vi "SinglePlaneScan.vi"(0 "Sweep Time (µS)":u32 step=2, 1 "Phase Shift (µS)":i32(slide) scale=-1000.0..1000.0, 2 "Sweep Interval (µS)":u32 step=2, 3 "Sample Rate (kHz)":u32, 4 "Offset":dbl, 5 "Amplitude":dbl) -> ()   [LabVIEW 2013]
doc: "I. Description:\nThis example demonstrates how to continuously acquire and generate data at the same time, synchronized with one another.\n\nII. Instructions for Running:\n1. Select the physical channel to correspond to where your signal is input on the DAQ device. Also, select the corresponding channel for where your signal is being generated.\n2. Enter the minimum and maximum voltage ranges.\nNote: For better accuracy try to match the input range to the expected voltage level of the measured signal.\n3. Set the sample rate of the acquisition.\nNote: The rate should be at least twice as fast as the maximum frequency component of the signal being acquired. \n6. Select the Rate for the generation\n7. Select what type of signal to generate and the amplitude.\nNote: This example requires two DMA channels to run. If your hardware does not support two DMA channels, you need to set the Data Transfer Mechanism property for the Analog Output Task to use \"Interrupts\". The Data Transfer Mechanism property is located in the DAQmx Channel Property hierarchy at:\n\nDAQmx Channel Property Node>>Analog Output>>General Properties>>Advanced>>Data Transfer and Memory>>Data Transfer Mechanism\n\nRefer to your device documentation to determine how many DMA channels are supported for your hardware.\n\nIII. Block Diagram Steps:\n1. Create an analog input voltage channel. Also, create an analog output voltage channel.\n2. Set the rate for the sample clock. Additionally, define the sample mode to be continuous. Also, set the sample clock rate for the signal generation.\n2a. Call the Get Terminal Name with Device Prefix VI. This will take a Task and a terminal and create a properly formatted device + terminal name to use as the source of the Trigger.\n3. Define the parameters for a Digital Edge Start Trigger. Set the Analog output to trigger off the AI Start Trigger. This is an internal trigger signal.\n4. Use the Basic Function Generator VI to create the signal to be generated.\n5. Call the Start VI to arm the two functions. Make sure the analog output is armed before the analog input. This will ensure both will start at the same time.\n6. Read the waveform data in a loop until the user hits the stop button or an error occurs. The Is Task Done? VI is used to check for errors in the Analog Output Task.\n7. Call the Clear VI to Clear the Task\n8. Use the popup dialog box to display an error if any.\n\nIV. I/O Connections Overview:\nMake sure your signal input/output terminals match the Physical Channel I/O controls."
uses:
  <vilib>/Utility/error.llb/DialogType.ctl
  <vilib>/DAQmx/write.llb/DAQmx Write (Analog Wfm 1Chan NSamp).vi
  <vilib>/DAQmx/write.llb/DAQmx Write (Digital 1D Wfm NChan NSamp).vi
  <vilib>/DAQmx/create/channels.llb/DAQmx Create Channel (CO-Pulse Generation-Time).vi
  <vilib>/DAQmx/create/channels.llb/DAQmx Create Channel (AO-Voltage-Basic).vi
  <vilib>/DAQmx/configure/timing.llb/DAQmx Timing (Sample Clock).vi
  <vilib>/DAQmx/create/channels.llb/DAQmx Create Channel (DO-Digital Output).vi
  <vilib>/DAQmx/configure/trigger.llb/DAQmx Start Trigger (Digital Edge).vi
  <vilib>/DAQmx/miscellaneous.llb/DAQmx Fill In Error Info.vi
  <vilib>/Waveform/DWDTOps.llb/DWDT Uncompress Digital.vi
panel:
  out "AOTF":digitalwaveform(graph)
  out "Resolution (µS)":u32
  out "Number of Samples":u32
  out "CAMERA EXPOSURE TRIGGER":digitalwaveform(graph)
  out "MIRROR":waveform(dbl)(graph)
  # "For instructions, select Help>>Show Context Help"
  # "Output Channel Parameters"
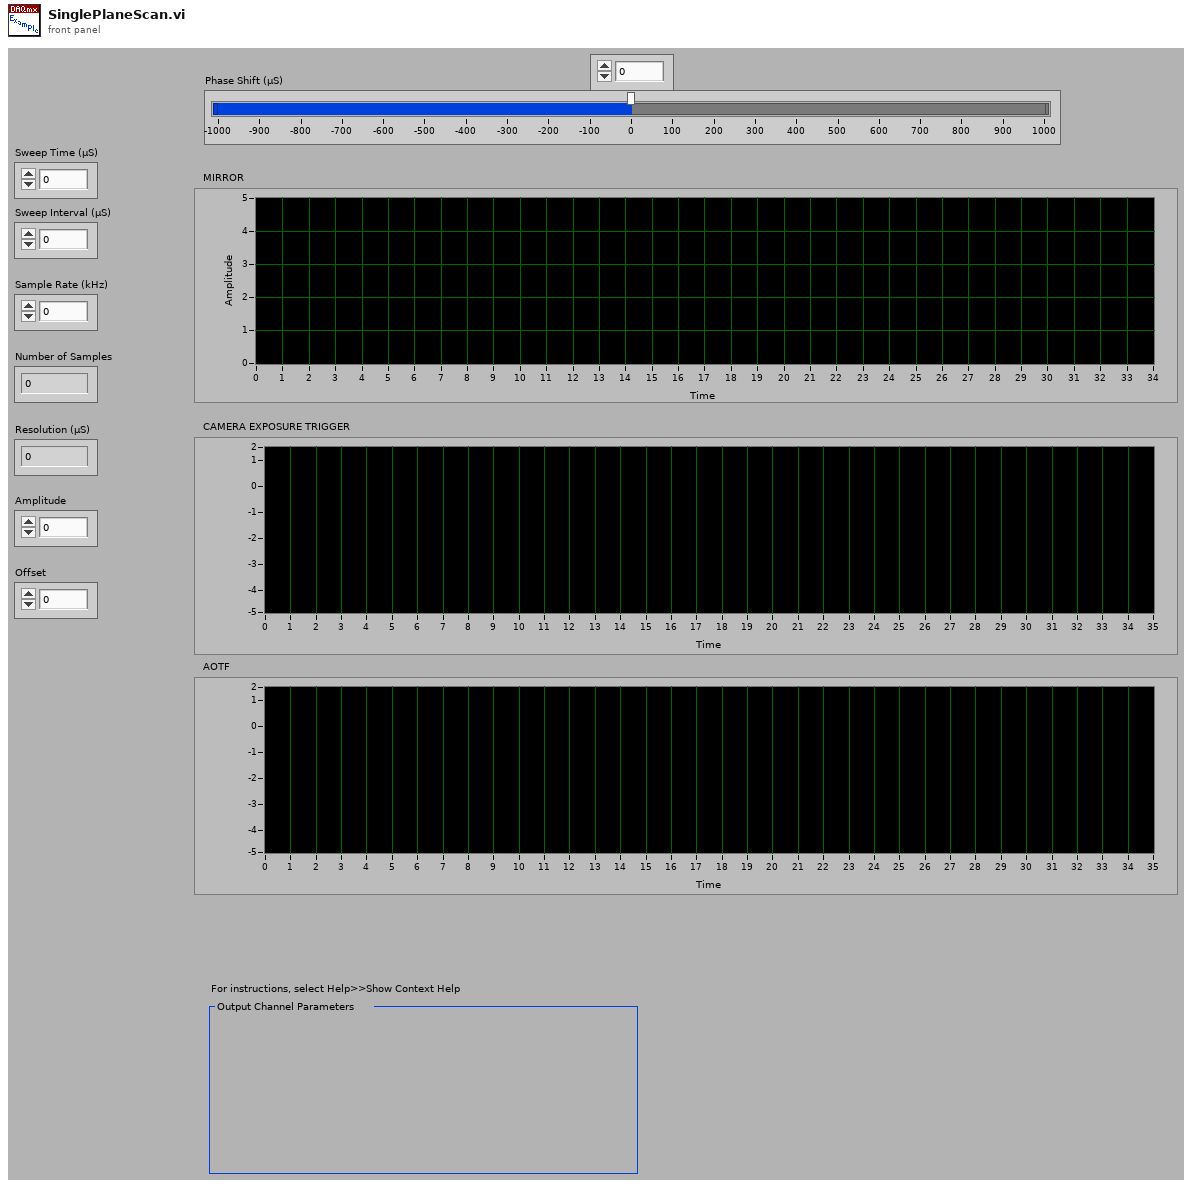
[diagram p1: front panel]
types:
  T1 = typedef "DialogType.ctl" = u16
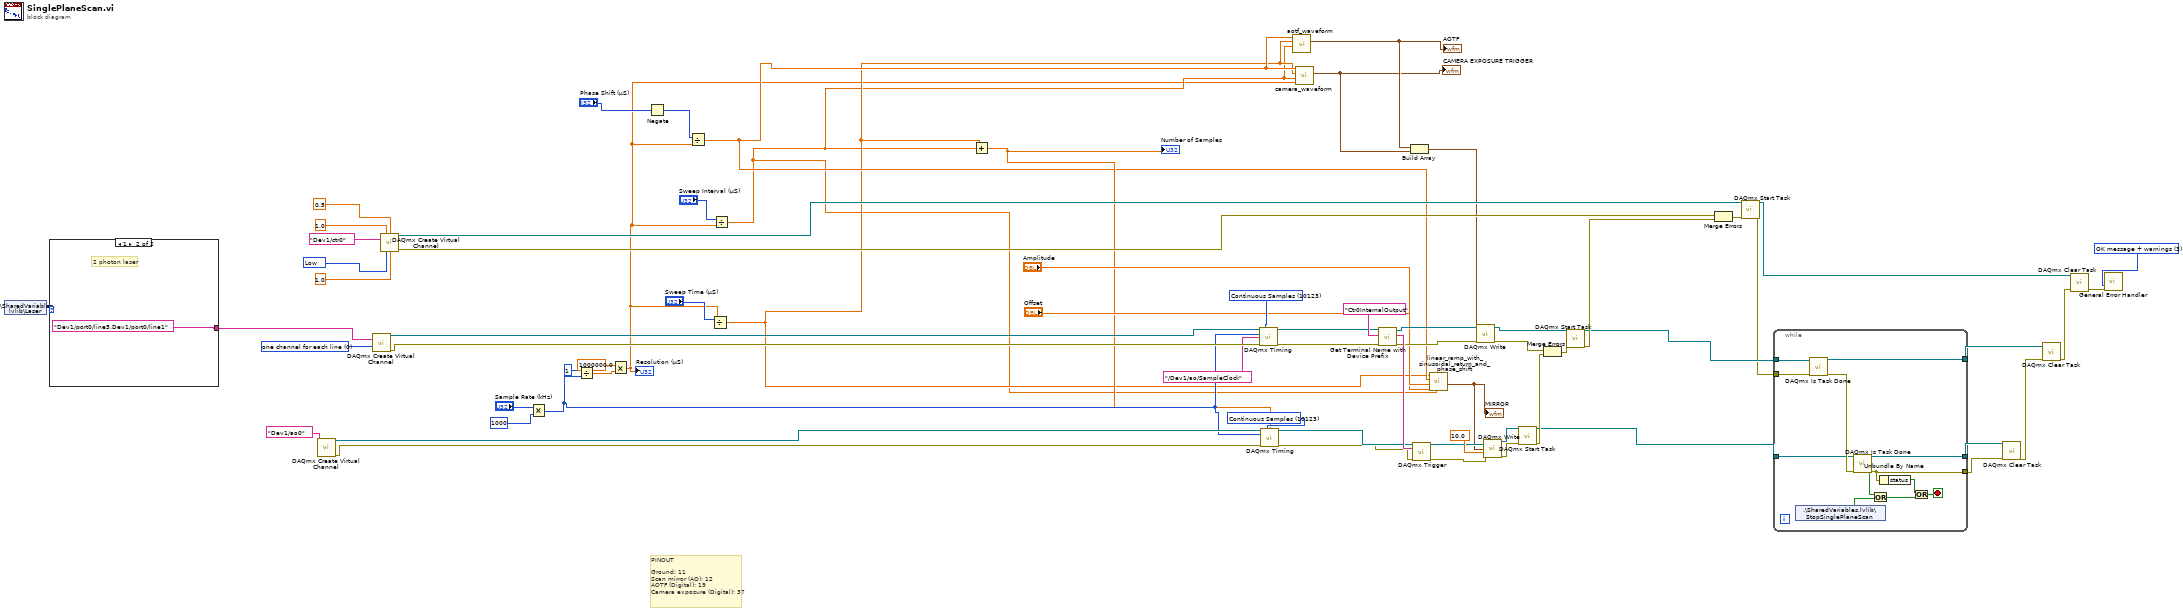
[diagram p0: block diagram]
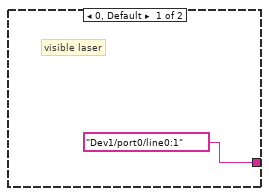
[diagram p2: hidden frame]
diagram:
  w25 = 0 items=["one channel for each line", "one channel for all lines"] ("line grouping")
  w36 = T1 3 items=["no dialog", "OK message", "continue or stop message", "OK message + warnings", "continue/stop + warnings"] ("type of dialog (OK msg:1)")
  w49 = 10214 items=["High"=10192, "Low"=10214] ("Idle State")
  w66 = 10123 items=["Finite Samples"=10178, "Continuous Samples"=10123] ("sample mode")
  w69 = 10123 items=["Finite Samples"=10178, "Continuous Samples"=10123] ("sample mode")
  # "PINOUT\n\nGround: 11\nScan mirror (AO): 12\nAOTF (Digital): 19\nCamera exposure (Digital): 37"
  n1 = shared-variable ".\\SharedVariables.lvlib\\Laser"() -> (w5:u8)  [unwired: 1 in, 1 out]
  n2 = case shown="1" w5 {
    tunnel: [tag "Dev1/port0/line0:1" ("Physical Channel") tag "Dev1/port0/line5,Dev1/port0/line1" ("Physical Channel")] -> w4
    frame 0, Default {
      # "visible laser"
    }
    frame 1 {
      # "2 photon laser"
    }
  }
  n3 = call-poly <vilib>:"DAQmx Create Virtual Channel.vi"("physical channels"=tag "Dev1/ao0") -> ("task out"=w65:refnum<k21>, "error out"=w64:errorcluster)  [unwired: 8 in, 5 out]
  n4 = call-poly <vilib>:"DAQmx Create Virtual Channel.vi"("lines"=w4, "line grouping"=w25) -> ("task out"=w67:refnum<k21>, "error out"=w68:errorcluster)  [unwired: 5 in, 7 out]
  n5 = call-poly <vilib>:"DAQmx Create Virtual Channel.vi"("high time"=1.0 ("High Time"), "low time"=0.5 ("Low Time"), "counter"=tag "Dev1/ctr0" ("Counter(s)"), "idle state"=w49, "initial delay"=1.0 ("Initial Delay")) -> ("task out"=w44:refnum<k21>, "error out"=w42:errorcluster)  [unwired: 4 in, 5 out]
  n6 = Multiply(x="Sample Rate (kHz)", y=u32 1000) -> (x*y=w15:u32)
  n7 = Divide(x=u32 1, y=w15) -> (x/y=w16:dbl)
  n8 = Multiply(x=1000000.0, y=w16) -> (x*y=w1:dbl)
  "Resolution (µS)" <- w1
  n9 = Negate(x="Phase Shift (µS)") -> (-x=w3:i32)
  n10 = Divide(x=w3, y=w1) -> (x/y=w10:dbl)
  n11 = Divide(x="Sweep Time (µS)", y=w1) -> (x/y=w9:dbl)
  n12 = Divide(x="Sweep Interval (µS)", y=w1) -> (x/y=w8:dbl)
  n13 = Add(x=w9, y=w8) -> (x+y=w12:dbl)
  "Number of Samples" <- w12
  n14 = call-poly <vilib>:"DAQmx Timing.vi"("task/channels in"=w67, "sample mode"=w69, "rate"=w15, "source"=tag "/Dev1/ao/SampleClock", "error in"=w68) -> ("task out"=w22:refnum<k21>, "error out"=w21:errorcluster)  [unwired: 2 in, 7 out]
  n15 = call-poly <vilib>:"DAQmx Timing.vi"("task/channels in"=w65, "sample mode"=w66, "samples per channel"=w12, "rate"=w15, "error in"=w64) -> ("task out"=w24:refnum<k21>, "error out"=w23:errorcluster)  [unwired: 2 in, 7 out]
  n16 = call "aotf_waveform.vi"("Sweep Interval (µS)"=w8, "Actual Sweep Time (µS)"=w9, "Phase Shift (µS)"=w10) -> ("Digital Waveform Graph"=w7:digitalwaveform)  [unwired: 8 in]
  "AOTF" <- w7
  n17 = call "camera_waveform.vi"("Resolution"=w1, "Sweep Interval (µS)"=w8, "Actual Sweep Time (µS)"=w9, "Phase Shift (µS)"=w10) -> ("Digital Waveform Graph"=w6:digitalwaveform)  [unwired: 7 in]
  "CAMERA EXPOSURE TRIGGER" <- w6
  n18 = call "Get Terminal Name with Device Prefix.vi"("error in (no error)"=w21, "Local Terminal Name"="Ctr0InternalOutput" ("terminal"), "task/channels in"=w22) -> ("error out"=w52:errorcluster, "Terminal Name with Device Prefix"=w57:tag, "task out"=w53:refnum<k21>)  [unwired: 1 in, 5 out]
  n19 = Build Array(w7, w6) -> (w26:digitalwaveform[])
  n20 = call-poly <vilib>:"DAQmx Trigger.vi"("task/channels in"=w24, "source"=w57, "error in"=w23) -> ("task out"=w59:refnum<k21>, "error out"=w60:errorcluster)  [unwired: 2 in, 9 out]
  n21 = call "linear_ramp_with_sinusoidal_return_and_phase_shift.vi"("Sweep Interval (µS)"=w8, "Offset"="Offset", "Amplitude"="Amplitude", "Phase Shift (µs)"=w10, "Sweep Time (µs)"=w9) -> ("Waveform Chart"=w27:waveform(dbl))  [unwired: 6 in]
  "MIRROR" <- w27
  n22 = call-poly <vilib>:"DAQmx Write.vi"("task/channels in"=w53, "data"=w26, "error in"=w52) -> ("task out"=w50:refnum<k21>, "error out"=w51:errorcluster)  [unwired: 2 in, 9 out]
  n23 = call-poly <vilib>:"DAQmx Write.vi"("task/channels in"=w59, "data"=w27, "timeout"=10.0 ("Wirite Timeout"), "error in"=w60) -> ("task out"=w62:refnum<k21>, "error out"=w61:errorcluster)  [unwired: 1 in, 9 out]
  n24 = call <vilib>:"DAQmx Start Task.vi"("task/channels in"=w62, "error in"=w61) -> ("task out"=w31:refnum<k21>, "error out"=w56:errorcluster)  [unwired: 12 out]
  n25 = Merge Errors(w51, w56) -> (w55:errorcluster)
  n26 = call <vilib>:"DAQmx Start Task.vi"("task/channels in"=w50, "error in"=w55) -> ("task out"=w30:refnum<k21>, "error out"=w43:errorcluster)  [unwired: 12 out]
  n27 = Merge Errors(w42, w43) -> (w41:errorcluster)
  n28 = call <vilib>:"DAQmx Start Task.vi"("task/channels in"=w44, "error in"=w41) -> ("task out"=w28:refnum<k21>, "error out"=w29:errorcluster)  [unwired: 12 out]
  n29 = while {
    tunnel: [w83] -> w38
    tunnel: w31 -> [w79]
    tunnel: [w78] -> w37
    tunnel: w30 -> [w77]
    tunnel: w29 -> [w76]
    tunnel: [w75] -> w35
    stop <- w82 stop-if-true
    n30 = shared-variable ".\\SharedVariables.lvlib\\StopSinglePlaneScan"() -> (w72:bool)  [unwired: 1 in, 1 out]
    n31 = call <vilib>:"DAQmx Is Task Done.vi"("task/channels in"=w77, "error in"=w76) -> ("task out"=w83:refnum<k21>, "error out"=w80:errorcluster)  [unwired: 2 in, 10 out]
    n32 = call <vilib>:"DAQmx Is Task Done.vi"("task/channels in"=w79, "error in"=w80) -> ("task out"=w78:refnum<k21>, "task done?"=w74:bool, "error out"=w75:errorcluster)  [unwired: 11 out]
    n33 = Or(x=w74, y=w72) -> (x .or. y?=w73:bool)
    n34 = Unbundle By Name(w75) -> ("status"=w81:bool)
    n35 = Or(x=w81, y=w73) -> (x .or. y?=w82:bool)
  }
  n36 = call <vilib>:"DAQmx Clear Task.vi"("task in"=w37, "error in"=w35) -> ("error out"=w34:errorcluster)  [unwired: 13 out]
  n37 = call <vilib>:"DAQmx Clear Task.vi"("task in"=w38, "error in"=w34) -> ("error out"=w33:errorcluster)  [unwired: 13 out]
  n38 = call <vilib>:"DAQmx Clear Task.vi"("task in"=w28, "error in"=w33) -> ("error out"=w32:errorcluster)  [unwired: 13 out]
  n39 = call <vilib>:"General Error Handler.vi"("type of dialog (OK msg:1)"=w36, "error in (no error)"=w32) -> ()  [unwired: 14 out]
